vi "ma_SML ND Zoom FFT Settings.vi"(6 "effective band specification":cluster{"fl":dbl, "fh":dbl}={"fl"=0.0, "fh"=0.5} {"fh" format="%.2f"; "fl" format="%.2f"}, 7 "RBW definition":enum16{"3dB", "6dB", "ENBW", "bin width"}(ring), 8 "error in (no error)":errorcluster, 9 "input signal type":enum16{"real", "complex modulated"}(ring), 10 "fs":dbl=1024.0 format="%.2f", 11 "spectrum settings":T1={"center frequency"=-inf, "span"=-1.0, "resolution bandwidth"=-1.0, "window"=0, "spectral lines"=-1} {"window" items=["Rectangle"=0, "Hanning"=1, "Hamming"=2, "Blackman-Harris"=3, "Exact Blackman"=4, "Blackman"=5, "Flat Top"=6, "4 Term B-Harris "=7, "7 Term B-Harris"=8, "Low Sidelobe"=9, "Blackman Nuttall"=11, "Triangle"=30, "Bartlett-Hanning"=31, "Bohman"=32, "Parzen"=33, "Welch"=34, "Kaiser"=60, "Dolph-Chebyshev"=61, "Gaussian"=62]; "resolution bandwidth" format="%.2f"; "center frequency" format="%.2f"; "span" format="%.2f"}) -> (0 "error out":errorcluster, 2 "zoom FFT settings":T2={"zoom settings"={"center frequency"=-inf, "zoom"=1, "trim"=1.0}, "FFT settings"={"window"=1, "FFT size"=-1}} {"FFT settings"."window" items=["Rectangle"=0, "Hanning"=1, "Hamming"=2, "Blackman-Harris"=3, "Exact Blackman"=4, "Blackman"=5, "Flat Top"=6, "4 Term B-Harris "=7, "7 Term B-Harris"=8, "Low Sidelobe"=9, "Blackman Nuttall"=11, "Triangle"=30, "Bartlett-Hanning"=31, "Bohman"=32, "Parzen"=33, "Welch"=34, "Kaiser"=60, "Dolph-Chebyshev"=61, "Gaussian"=62]; "zoom settings"."trim" min=1.0 format="%.2f"; "zoom settings"."center frequency" format="%.2f"; "zoom settings"."zoom" min=1}, 3 "actual spectrum settings":T1={"center frequency"=-inf, "span"=-1.0, "resolution bandwidth"=-1.0, "window"=0, "spectral lines"=-1} {"window" items=["Rectangle"=0, "Hanning"=1, "Hamming"=2, "Blackman-Harris"=3, "Exact Blackman"=4, "Blackman"=5, "Flat Top"=6, "4 Term B-Harris "=7, "7 Term B-Harris"=8, "Low Sidelobe"=9, "Blackman Nuttall"=11, "Triangle"=30, "Bartlett-Hanning"=31, "Bohman"=32, "Parzen"=33, "Welch"=34, "Kaiser"=60, "Dolph-Chebyshev"=61, "Gaussian"=62]; "resolution bandwidth" format="%.2f"; "center frequency" format="%.2f"; "span" format="%.2f"}, 5 "aquisition size":i32)   [LabVIEW 2020, in "NI_MAPro.lvlib"]
uses:
  NI_MAPro.lvlib
  ma_sml_BZ Spectrum Settings.ctl
  ma_sml_ND Zoom FFT Settings.ctl
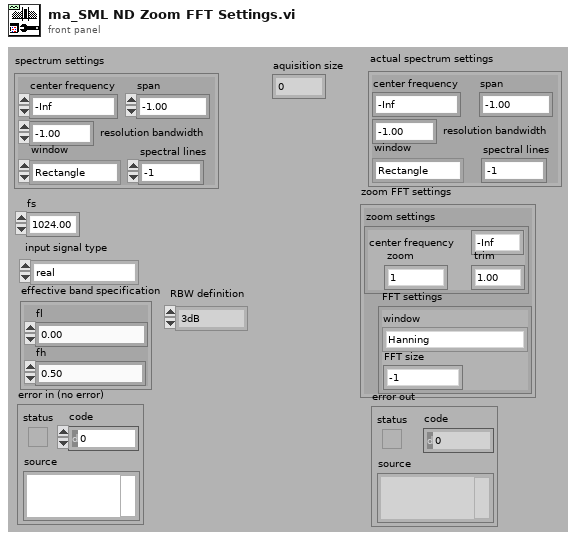
[diagram p1: front panel]
types:
  T1 = typedef "NI_MAPro.lvlib/ma_sml_BZ Spectrum Settings.ctl" = cluster{"center frequency":dbl, "span":dbl, "resolution bandwidth":dbl, "window":u16, "spectral lines":i32}
  T2 = typedef "NI_MAPro.lvlib/ma_sml_ND Zoom FFT Settings.ctl" = cluster{"zoom settings":cluster{"center frequency":dbl, "zoom":i32, "trim":dbl}, "FFT settings":cluster{"window":u16, "FFT size":i32}}
  T3 = cluster{"aquisition size":i32, "actual RBW":dbl, "zoom FFT settings":T2}
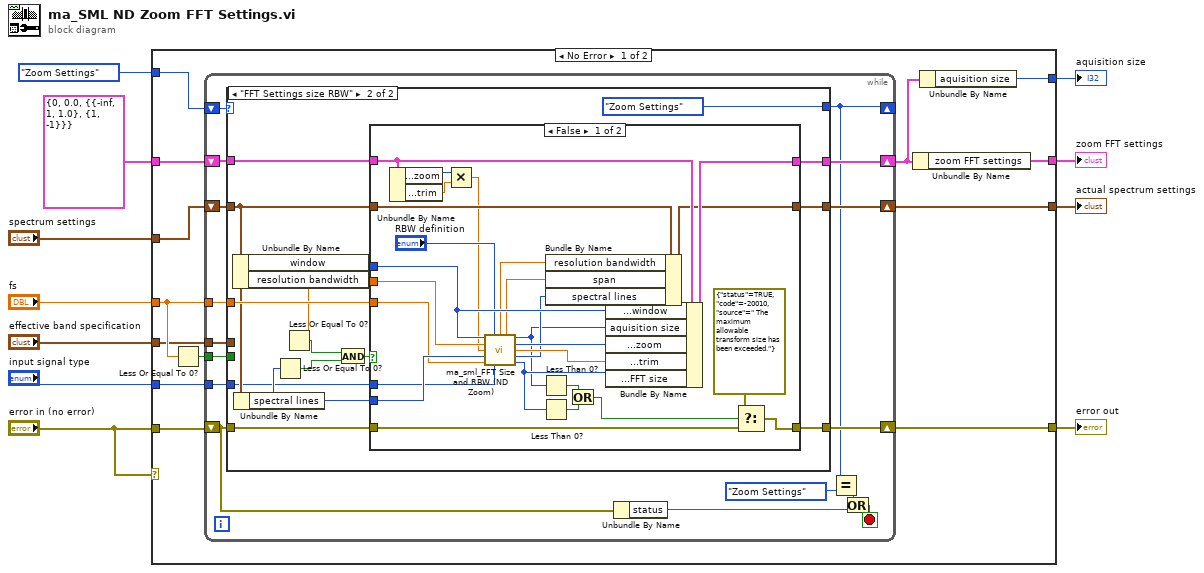
[diagram p0: block diagram]
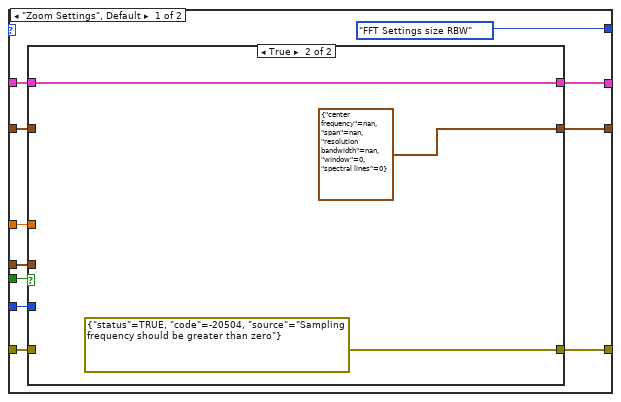
[diagram p2: hidden frame]
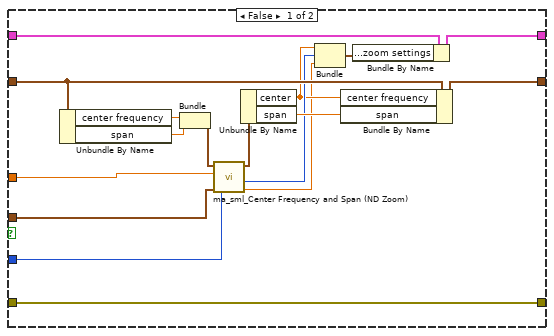
[diagram p3: hidden frame]
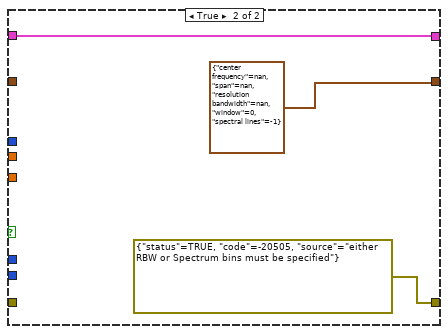
[diagram p4: hidden frame]
diagram:
  n1 = case shown="No Error" "error in (no error)" {
    tunnel: "error in (no error)" -> [w24 w116]
    tunnel: [w23 w116] -> w11
    tunnel: [w20 _] -> w9
    tunnel: [w19 _] -> w8
    tunnel: [w18 _] -> w7
    tunnel: "spectrum settings" -> [w17 _]
    tunnel: "fs" -> [w16 _]
    tunnel: "effective band specification" -> [w15 _]
    tunnel: "input signal type" -> [w14 _]
    tunnel: T3 {"aquisition size"=0, "actual RBW"=0.0, "zoom FFT settings"={"zoom settings"={"center frequency"=-inf, "zoom"=1, "trim"=1.0}, "FFT settings"={"window"=1, "FFT size"=-1}}} -> [w13 _]
    tunnel: enum16{"Zoom Settings", "FFT Settings size RBW"}."Zoom Settings" -> [w12 _]
    frame No Error {
      n2 = Less Or Equal To 0?(x=w16) -> (x <= 0?=w21:bool)
      n3 = while {
        tunnel: w15 -> [w25]
        tunnel: w14 -> [w26]
        tunnel: w21 -> [w27]
        shift-left: w17 -> [w32]
        shift-right: [w31] -> w18
        shift-left: w24 -> [w35]
        shift-right: [w34] -> w23
        shift-left: w12 -> [w30]
        shift-right: [w29] -> _
        shift-left: w13 -> [w39]
        shift-right: [w33] -> w22
        tunnel: w16 -> [w40]
        stop <- w36 stop-if-true
        n4 = case shown="\"FFT Settings size RBW\"" w30 {
          tunnel: w40 -> [w50 w81]
          tunnel: w39 -> [w44 w80]
          tunnel: [w43 w79] -> w33
          tunnel: w35 -> [w46 w84]
          tunnel: [w45 w83] -> w34
          tunnel: [enum16{"Zoom Settings", "FFT Settings size RBW"}."FFT Settings size RBW" enum16{"Zoom Settings", "FFT Settings size RBW"}."Zoom Settings"] -> w29
          tunnel: w32 -> [w49 w78]
          tunnel: [w48 w77] -> w31
          tunnel: w27 -> [w47 _]
          tunnel: w26 -> [w42 w75]
          tunnel: w25 -> [w41 _]
          frame "Zoom Settings", Default {
            n5 = case shown="True" w47 {
              tunnel: w50 -> [w63 _]
              tunnel: w49 -> [w66 _]
              tunnel: [w68 T1 {"center frequency"=nan, "span"=nan, "resolution bandwidth"=nan, "window"=0, "spectral lines"=0} ("actual spectrum settings")] -> w48
              tunnel: [w67 errorcluster {"status"=TRUE, "code"=-20504, "source"="Sampling frequency should be greater than zero"} ("error in (no error)")] -> w45
              tunnel: w46 -> [w67 _]
              tunnel: w44 -> [w59 w70]
              tunnel: [w60 w70] -> w43
              tunnel: w42 -> [w58 _]
              tunnel: w41 -> [w53 _]
              frame False {
                n6 = Unbundle By Name(w66) -> ("center frequency"=w65:dbl, "span"=w54:dbl)
                n7 = Bundle("center frequency"=w65, "span"=w54) -> (w64:cluster{"center frequency":dbl, "span":dbl})  [unwired: 1 out]
                n8 = call "ma_sml_Center Frequency and Span (ND Zoom).vi"("effective band specification"=w53, "input signal type"=w58, "fs"=w63, "desired center span"=w64) -> ("trim"=w52:dbl, "zoom"=w57:i32, "actual center span"=w62:cluster{"center":dbl, "span":dbl})  [unwired: 1 out]
                n9 = Unbundle By Name(w62) -> ("center"=w56:dbl, "span"=w61:dbl)
                n10 = Bundle("center"=w56, "zoom"=w57, "trim"=w52) -> (w55:cluster{"center":dbl, "zoom":i32, "trim":dbl})  [unwired: 1 out]
                n11 = Bundle By Name(cluster=w66, "center frequency"=w56, "span"=w61) -> (w68:T1)
                n12 = Bundle By Name(cluster=w59, "zoom FFT settings.zoom settings"=w55) -> (w60:T3)
              }
              frame True {
              }
            }
          }
          frame "FFT Settings size RBW" {
            n13 = Unbundle By Name(w78) -> ("window"=w82:u16, "resolution bandwidth"=w72:dbl)
            n14 = Unbundle By Name(w78) -> ("spectral lines"=w86:i32)
            n15 = Less Or Equal To 0?(x=w86) -> (x <= 0?=w73:bool)
            n16 = Less Or Equal To 0?(x=w72) -> (x <= 0?=w74:bool)
            n17 = And(x=w74, y=w73) -> (x .and. y?=w85:bool)
            n18 = case shown="False" w85 {
              tunnel: w84 -> [w90 _]
              tunnel: [w89 errorcluster {"status"=TRUE, "code"=-20505, "source"="either RBW or Spectrum bins must be specified"} ("error in (no error)")] -> w83
              tunnel: w82 -> [w103 _]
              tunnel: w81 -> [w104 _]
              tunnel: w80 -> [w112 w114]
              tunnel: w86 -> [w106 _]
              tunnel: [w111 w114] -> w79
              tunnel: w78 -> [w110 _]
              tunnel: [w109 T1 {"center frequency"=nan, "span"=nan, "resolution bandwidth"=nan, "window"=0, "spectral lines"=-1} ("spectrum settings")] -> w77
              tunnel: w72 -> [w108 _]
              tunnel: w75 -> [w105 _]
              frame False {
                n19 = Unbundle By Name(w112) -> ("zoom FFT settings.zoom settings.zoom"=w107:i32, "zoom FFT settings.zoom settings.trim"=w97:dbl)
                n20 = Multiply(x=w107, y=w97) -> (x*y=w98:dbl)
                n21 = call "ma_sml_FFT Size and RBW (ND Zoom).vi"("window"=w103, "RBW definition"="RBW definition", "RBW"=w108, "zoom"=w98, "spectral lines"=w106, "fs"=w104, "input signal type"=w105) -> ("RBW actual"=w102:dbl, "span"=w101:dbl, "acq. size"=w87:i32, "zoom factor"=w100:i32, "trimming factor"=w96:dbl, "spectral lines actual"=w95:i32, "FFT Size"=w94:i32)  [unwired: 2 out]
                n22 = Less Than 0?(x=w87) -> (x < 0?=w93:bool)
                n23 = Less Than 0?(x=w94) -> (x < 0?=w92:bool)
                n24 = Bundle By Name(cluster=w110, "resolution bandwidth"=w102, "span"=w101, "spectral lines"=w95) -> (w109:T1)
                n25 = Or(x=w93, y=w92) -> (x .or. y?=w91:bool)
                n26 = Bundle By Name(cluster=w112, "zoom FFT settings.FFT settings.window"=w103, "aquisition size"=w87, "zoom FFT settings.zoom settings.zoom"=w100, "zoom FFT settings.zoom settings.trim"=w96, "zoom FFT settings.FFT settings.FFT size"=w94) -> (w111:T3)
                n27 = Select(t=errorcluster {"status"=TRUE, "code"=-20010, "source"=" The maximum allowable transform size has been exceeded."}, s=w91, f=w90) -> (s? t:f=w89:errorcluster)
              }
              frame True {
              }
            }
          }
        }
        n28 = Unbundle By Name(w35) -> ("status"=w37:bool)
        n29 = Equal?(x=w29, y=enum16{"Zoom Settings", "FFT Settings size RBW"}."Zoom Settings") -> (x = y?=w38:bool)
        n30 = Or(x=w38, y=w37) -> (x .or. y?=w36:bool)
      }
      n31 = Unbundle By Name(w22) -> ("zoom FFT settings"=w19:T2)
      n32 = Unbundle By Name(w22) -> ("aquisition size"=w20:i32)
    }
    frame Error {
    }
  }
  "error out" <- w11
  "aquisition size" <- w9
  "zoom FFT settings" <- w8
  "actual spectrum settings" <- w7
